vi "DECODIFICAR ESTADO PUERTO.vi"(11 "ESTADO DEL PUERTO":string) -> (3 "Array":bool[](array[boolean]))   [LabVIEW 2019]
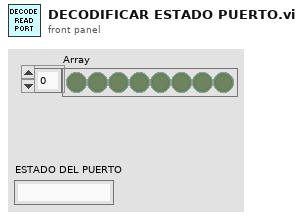
[diagram p1: front panel]
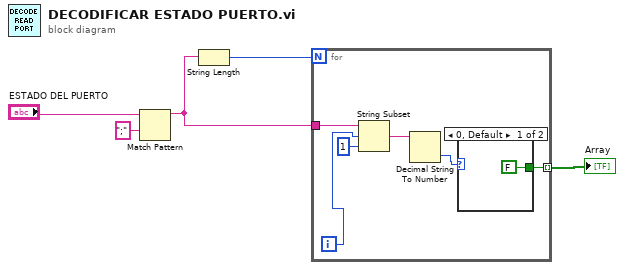
[diagram p0: block diagram]
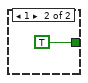
[diagram p2: hidden frame]
diagram:
  n1 = Match Pattern(string="ESTADO DEL PUERTO", regular expression=";") -> (before substring=w2:string)  [unwired: 1 in, 3 out]
  n2 = String Length(string=w2) -> (length=w3:i32)
  n3 = for {
    N: w3 -> [_]
    tunnel: w2 -> [w11]
    tunnel: [w6] -> w1 mode=indexing
    i -> [w9]
    n4 = String Subset(string=w11, offset (0)=w9, length (rest)=1 ("length (rest)")) -> (substring=w8:string)
    n5 = Decimal String To Number(string=w8) -> (number=w7:i32)  [unwired: 2 in, 1 out]
    n6 = case shown="0, Default" w7 {
      tunnel: [FALSE TRUE] -> w6
      frame 0, Default {
      }
      frame 1 {
      }
    }
  }
  "Array" <- w1
